vi "Constructor-Port.vi"(8 "error in (no error)":errorcluster, 11 "ListenerPort":u16) -> (0 "error out":errorcluster, 3 "ServiceManager out":refnum<class "ServiceManager.lvclass">)   [LabVIEW 2020, in "ServiceManager.lvlib" / "ServiceManager.lvclass"]
uses:
  ServiceManager.lvclass
  ServiceManager.lvclass/ServiceManager.ctl
panel:
  in  "DebugView":bool
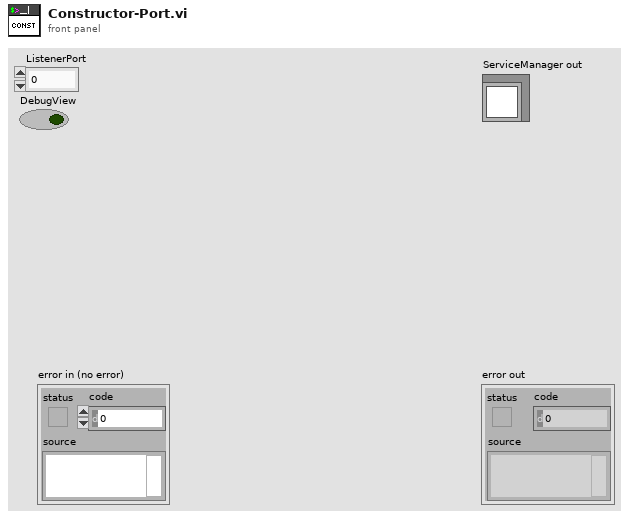
[diagram p1: front panel]
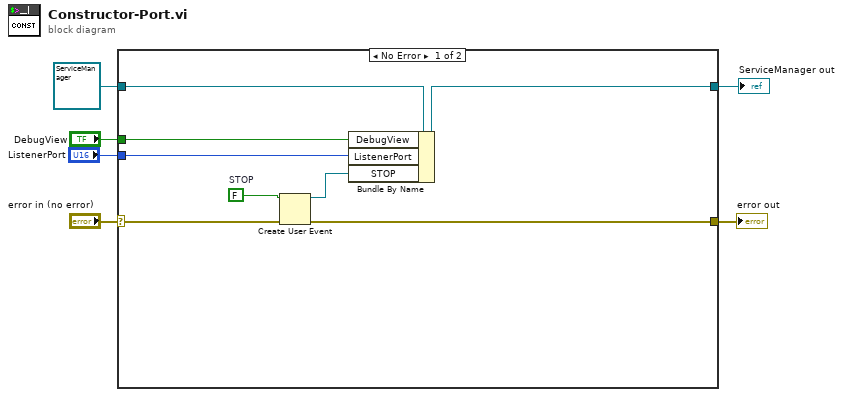
[diagram p0: block diagram]
diagram:
  n1 = case shown="No Error" "error in (no error)" {
    selector: "error in (no error)" -> [w11 w16]
    tunnel: [w10 w16] -> w5
    tunnel: [w13 w15] -> w3
    tunnel: refnum<class "ServiceManager.lvclass"> refnum ("ServiceManager in") -> [w14 w15]
    tunnel: "ListenerPort" -> [w12 _]
    tunnel: "DebugView" -> [w7 _]
    frame No Error {
      w9 = FALSE  # STOP
      n2 = Create User Event(user event datatype=w9, error in=w11) -> (user event=w8:refnum<user-event>, error out=w10:errorcluster)
      n3 = Bundle By Name(cluster=w14, "DebugView"=w7, "ListenerPort"=w12, "STOP"=w8) -> (w13:refnum<class "ServiceManager.lvclass">)
    }
    frame Error {
    }
  }
  "error out" <- w5
  "ServiceManager out" <- w3
